vi "cameraSetup.vi"() -> ()   [LabVIEW 2024]
uses:
  <vilib>/userDefined/High Color/IMAQdx.ctl
  <vilib>/Python/Open Venv Python Session.vi
  <vilib>/vision/NI_Vision_Development_Module.lvlib
  <vilib>/vision/driver/NI_Vision_Acquisition_Software.lvlib
panel:
  out "Python Node Process Time":dbl
  out "error out":errorcluster
  out "PointCloud":T1(graph)=[{"appended array"=[-1.3170576278200137, -1.3344662442040491, -1.3432764589201578, -1.3444474689182773, -1.338872970131032, -1.327383409908652, -1.3107482394539027, -1.289678166257004, -1.26482740653056, -1.2367959376444793, -1.206131750560902, -1.1733331022691227, -1.1388507682205156, -1.1030902947634595, -1.0664142515782609, -1.0291444841120803, -0.9915643660138534, -0.9539210515692201, -0.9164277281354453, -0.879265868576345, -0.8425874836972105, -0.8065173746797322, -0.7711553855169254, -0.7365786554480533, -0.7028438713935529, -0.6699895203899575, -0.6380381420248239, -0.6069985808716541, -0.5768682389248215, -0.5476353280344943, -0.5192811223415612, -0.49178221071255507, -0.46511274917457684, -0.439246713350222, -0.41416015089250097, -0.38983343391976977, -0.3662535114506477, -0.34341616183894813, -0.3213282452085969, -0.300009955888562, -0.27949707484777436, -0.259843222130055, -0.2411221092890378, -0.22342979182309308, -0.2068869216102553, -0.19164099934314494, -0.17786862696389336, -0.16577776009906756, -0.15560996049459447, -0.14764264845068567], "appended array"=[0.03, 0.09530612244897953, 0.16061224489795906, 0.22591836734693857, 0.2912244897959181, 0.3565306122448982, 0.4218367346938777, 0.4871428571428572, 0.5524489795918368, 0.6177551020408163, 0.6830612244897958, 0.7483673469387756, 0.8136734693877551, 0.8789795918367347, 0.9442857142857145, 1.0095918367346939, 1.0748979591836736, 1.140204081632653, 1.2055102040816326, 1.2708163265306123, 1.336122448979592, 1.4014285714285715, 1.4667346938775512, 1.5320408163265307, 1.5973469387755104, 1.6626530612244899, 1.7279591836734693, 1.793265306122449, 1.8585714285714285, 1.9238775510204082, 1.989183673469388, 2.0544897959183674, 2.119795918367347, 2.1851020408163264, 2.250408163265306, 2.315714285714286, 2.3810204081632653, 2.446326530612245, 2.5116326530612247, 2.5769387755102042, 2.6422448979591837, 2.707551020408163, 2.7728571428571427, 2.838163265306122, 2.9034693877551025, 2.968775510204082, 3.0340816326530615, 3.099387755102041, 3.1646938775510205, 3.23]}, {"appended array"=[1.1959745945438647, 1.1539974976878962, 1.116034957811131, 1.081567752911547, 1.050122782354486, 1.021271082137672, 0.9946258401561943, 0.9698404114675151, 0.9466063335564582, 0.9246513416002126, 0.9037373837333251, 0.8836586363127031, 0.8642395191826058, 0.8453327109396446, 0.8268171641977818, 0.8085961208533234, 0.7905951273499227, 0.7727600499435693, 0.7550550899675955, 0.737460799097667, 0.7199720946167827, 0.702596274680272, 0.6853510335807903, 0.6682624770133202, 0.6513631373401643, 0.6346899888559443, 0.6182824630525999, 0.6021804638843833, 0.5864223830328587, 0.5710431151718984, 0.5560720732326803, 0.5415312036686851, 0.5274330017206939, 0.5137785266817849, 0.5005554171623322, 0.4877359063550006, 0.4752748372997456, 0.46310767814880766, 0.45114853743171296, 0.43928817932026787, 0.4273920388935579, 0.41529823740294264, 0.40281559753705665, 0.38972165868680464, 0.3757606922103577, 0.36064171669815265, 0.34403651323788836, 0.32557764067952294, 0.3048564509002722, 0.2814211040696046], "appended array"=[0.07, 0.13530612244897952, 0.20061224489795904, 0.2659183673469386, 0.3312244897959181, 0.39653061224489816, 0.4618367346938777, 0.5271428571428572, 0.5924489795918367, 0.6577551020408163, 0.7230612244897958, 0.7883673469387756, 0.8536734693877551, 0.9189795918367346, 0.9842857142857144, 1.049591836734694, 1.1148979591836736, 1.1802040816326531, 1.2455102040816326, 1.3108163265306123, 1.3761224489795918, 1.4414285714285715, 1.5067346938775512, 1.5720408163265307, 1.6373469387755102, 1.70265306122449, 1.7679591836734694, 1.833265306122449, 1.8985714285714286, 1.9638775510204083, 2.029183673469388, 2.0944897959183675, 2.159795918367347, 2.2251020408163265, 2.290408163265306, 2.355714285714286, 2.4210204081632654, 2.486326530612245, 2.5516326530612248, 2.6169387755102043, 2.6822448979591837, 2.7475510204081632, 2.8128571428571427, 2.878163265306122, 2.9434693877551026, 3.008775510204082, 3.0740816326530616, 3.139387755102041, 3.2046938775510205, 3.27]}, {"appended array"=[-2.1976754604858093, -2.1730091080730474, -2.147243328942704, -2.120370792552189, -2.0923975746039645, -2.063342224625402, -2.033234833548644, -2.002116101290463, -1.9700364043321177, -1.937054863299217, -1.903238410541575, -1.86866085771307, -1.8334019633515066, -1.7975465004584736, -1.7611833240791992, -1.7244044388824187, -1.687304066740224, -1.6499777143079288, -1.6125212406039253, -1.5750299245895452, -1.5375975327489153, -1.5003153866688206, -1.4632714306185601, -1.426549299129809, -1.3902273845764739, -1.3543779047545552, -1.3190659704620058, -1.284348653078588, -1.250274052145734, -1.216880362946406, -1.1841949440849537, -1.1522333850669733, -1.1209985738791681, -1.0904797645692061, -1.0606516448255798, -1.031473403557465, -1.0028877984745799, -0.9748202236670446, -0.9471777771852397, -0.9198483286196648, -0.8926995866807996, -0.8655781667789612, -0.8383086586041626, -0.810692693705974, -0.7825080130733804, -0.7535075347146409, -0.7234184212371477, -0.6919411474272857, -0.6587485678302909, -0.6234849843301098], "appended array"=[0.12, 0.18428571428571444, 0.24857142857142833, 0.3128571428571428, 0.3771428571428572, 0.44142857142857167, 0.5057142857142856, 0.5700000000000001, 0.6342857142857145, 0.698571428571429, 0.7628571428571428, 0.8271428571428573, 0.8914285714285715, 0.9557142857142855, 1.02, 1.0842857142857145, 1.1485714285714286, 1.2128571428571429, 1.2771428571428574, 1.3414285714285716, 1.405714285714286, 1.47, 1.5342857142857145, 1.5985714285714288, 1.6628571428571428, 1.7271428571428573, 1.7914285714285714, 1.8557142857142859, 1.92, 1.9842857142857144, 2.0485714285714285, 2.112857142857143, 2.1771428571428575, 2.2414285714285715, 2.305714285714286, 2.37, 2.4342857142857146, 2.4985714285714287, 2.5628571428571436, 2.6271428571428572, 2.6914285714285717, 2.755714285714286, 2.82, 2.8842857142857143, 2.948571428571429, 3.012857142857143, 3.0771428571428574, 3.141428571428572, 3.2057142857142855, 3.27]}, {"appended array"=[2.0462614612009418, 2.012322089098866, 1.9811875610569154, 1.9523916760385782, 1.9255095718547126, 1.9001560984615924, 1.8759841912589486, 1.8526832443880148, 1.8299774840295686, 1.8076243417019748, 1.7854128275592256, 1.7631619036889907, 1.7407188574106534, 1.7179576745733556, 1.6947774128540425, 1.6711005750555046, 1.646871482404418, 1.6220546478493925, 1.5966331493590098, 1.5706070032198705, 1.5439915373346338, 1.516815764520062, 1.4891207558050628, 1.4609580137287332, 1.4323878456384034, 1.4034777369876759, 1.3743007246344723, 1.3449337701390756, 1.315456133062171, 1.2859477442628913, 1.2564875791968586, 1.2271520312142292, 1.198013284857733, 1.1691376891607195, 1.140584130945199, 1.1124024081198882, 1.0846316029782503, 1.0572984554965381, 1.03041573663184, 1.003980621620119, 0.9779730632742587, 0.9523541652821047, 0.9270645555045082, 0.9020227592733693, 0.8771235726896788, 0.8522364359215618, 0.8272038065023218, 0.8018395326284821, 0.7759272264578283, 0.7492186374074544], "appended array"=[0.32, 0.380204081632653, 0.440408163265306, 0.5006122448979591, 0.5608163265306121, 0.6210204081632651, 0.6812244897959181, 0.7414285714285714, 0.8016326530612244, 0.8618367346938777, 0.9220408163265308, 0.9822448979591838, 1.0424489795918368, 1.1026530612244898, 1.1628571428571428, 1.2230612244897958, 1.2832653061224488, 1.3434693877551018, 1.403673469387755, 1.463877551020408, 1.5240816326530613, 1.5842857142857145, 1.6444897959183673, 1.7046938775510205, 1.7648979591836735, 1.8251020408163265, 1.8853061224489795, 1.9455102040816326, 2.005714285714286, 2.065918367346939, 2.126122448979592, 2.186326530612245, 2.246530612244898, 2.306734693877551, 2.366938775510204, 2.427142857142857, 2.4873469387755103, 2.5475510204081635, 2.6077551020408163, 2.6679591836734695, 2.7281632653061223, 2.7883673469387755, 2.8485714285714288, 2.9087755102040815, 2.9689795918367343, 3.029183673469388, 3.089387755102041, 3.149591836734694, 3.2097959183673472, 3.27]}]
  out "Image":T2(plugin-control)
  out "yellow_right_y":dbl[](array[numeric])
  out "yellow_right_x":dbl[](array[numeric])
  out "yellow_left_y":dbl[](array[numeric])
  out "yellow_left_x":dbl[](array[numeric])
  out "white_right_y":dbl[](array[numeric])
  out "white_right_x":dbl[](array[numeric])
  out "white_left_y":dbl[](array[numeric])
  out "white_left_x":dbl[](array[numeric])
  in  "Test":bool=TRUE
  in  "Cam No.":T3
  out "Python Loop Process Time":u32=101
  out "B Pixels":u8[][](array[numeric])
  out "G Pixels":u8[][](array[numeric])
  out "R Pixels":u8[][](array[numeric])
  out "Image2Array LoopTime":u32=101
  in  "stop":bool
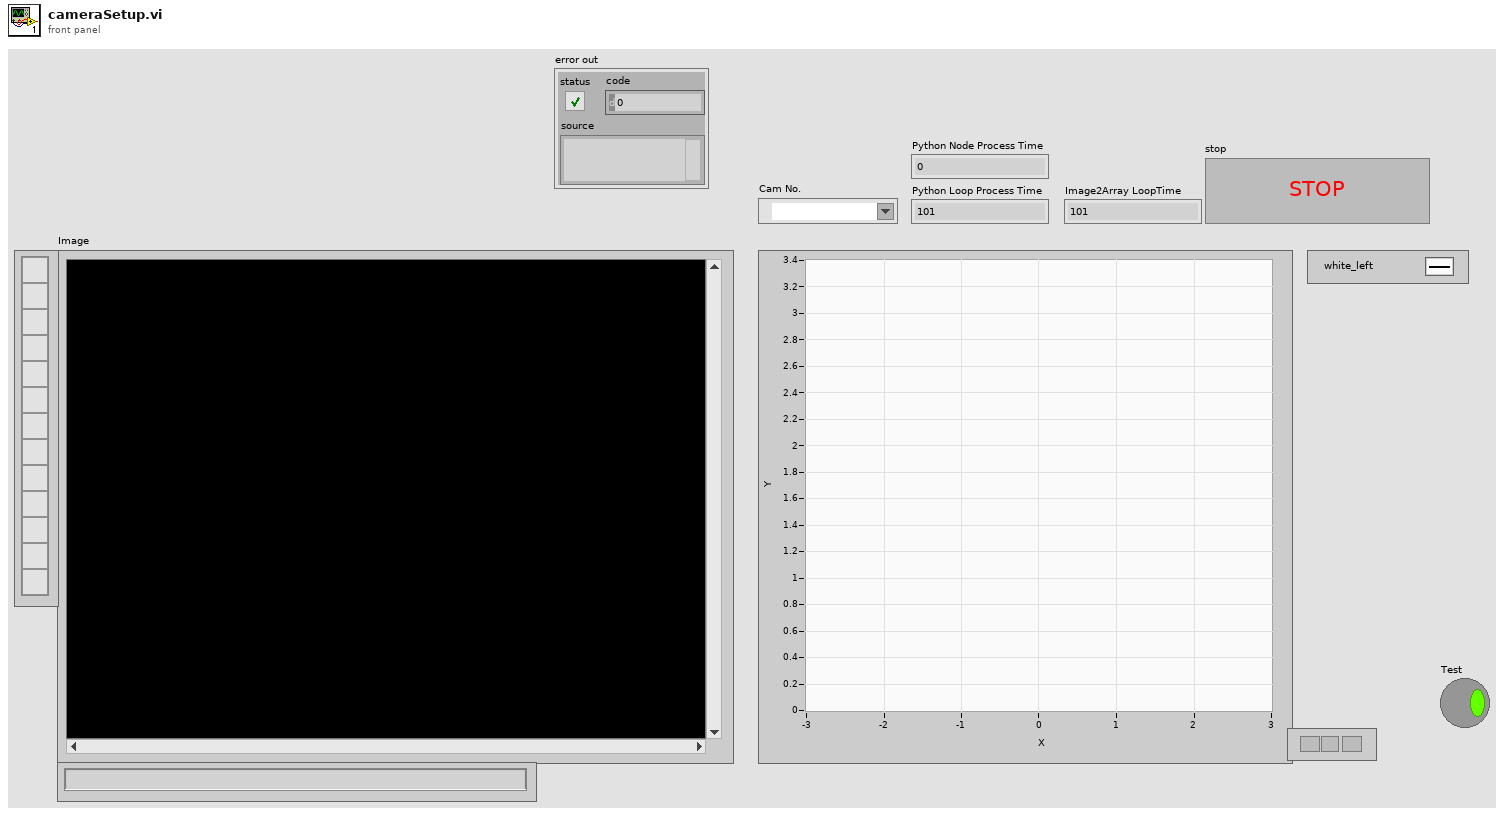
[diagram p1: front panel]
types:
  T1 = cluster{"appended array":dbl[], "appended array":dbl[]}[]
  T2 = typedef "IMAQ Image.ctl" = refnum<image>
  T3 = typedef "IMAQdx.ctl" = refnum<k21>
  T4 = cluster{"white_left_x":dbl[], "white_left_y":dbl[]}
  T5 = cluster{"white_right_x":dbl[], "white_right_y":dbl[]}
  T6 = cluster{"yellow_left_x":dbl[], "yellow_left_y":dbl[]}
  T7 = cluster{"yellow_right_x":dbl[], "yellow_right_y":dbl[]}
  T8 = cluster{"yellow_right_x":dbl[], "yellow_right_y":dbl[]}[]
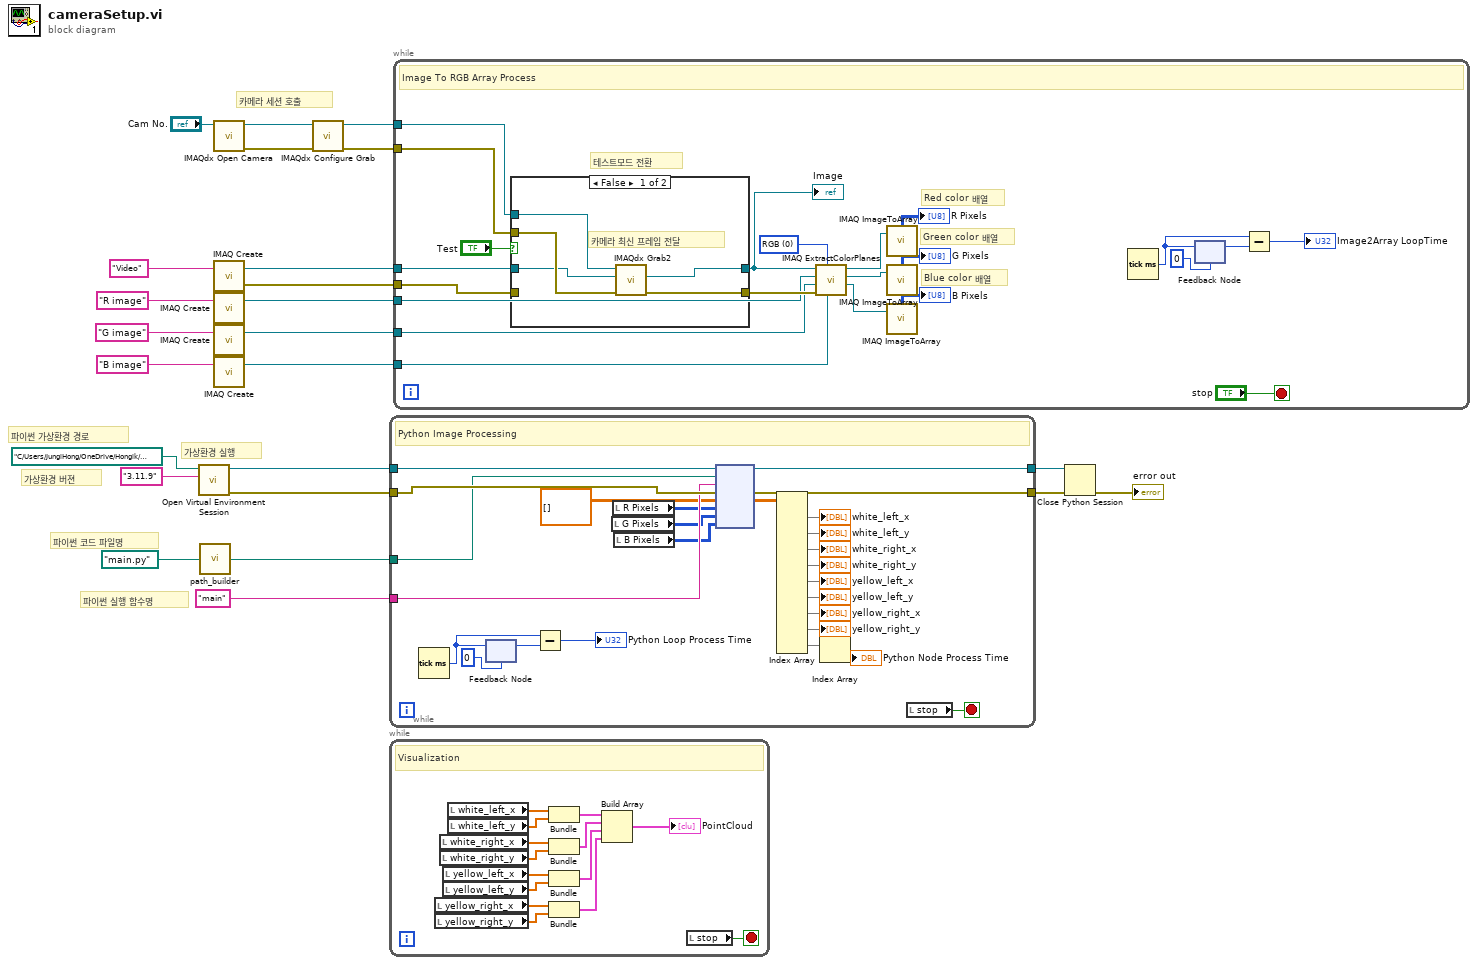
[diagram p0: block diagram]
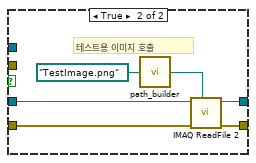
[diagram p2: hidden frame]
diagram:
  # "파이썬 실행 함수명"
  # "파이썬 코드 파일명"
  # "가상환경 실행"
  # "가상환경 버젼"
  # "파이썬 가상환경 경로"
  # "카메라 세션 호출"
  n1 = call-poly <vilib>:"Open Virtual Environment Session.vi"("Python version"="3.11.9", "Env path"=path "C:/Users/JungiHong/OneDrive/Hongik/HI-RACE/2026-01/.venv") -> ("error out"=w10:errorcluster, "session out"=w11:refnum<k35>)  [unwired: 8 in]
  n2 = call "path_builder.vi"("Name"=path "main.py") -> ("appended path"=w9:path)
  n3 = call <vilib>:"IMAQdx Open Camera.vi"("Session In"="Cam No.") -> ("error out"=w5:errorcluster, "Session Out"=w6:T3)  [unwired: 9 in]
  n4 = call "IMAQ Create"("Image Name"="Video") -> ("New Image"=w20:T2, "error out"=w21:errorcluster)  [unwired: 4 in]
  n5 = call "IMAQ Create"("Image Name"="R image") -> ("New Image"=w16:T2)  [unwired: 4 in, 1 out]
  n6 = call "IMAQ Create"("Image Name"="G image") -> ("New Image"=w15:T2)  [unwired: 4 in, 1 out]
  n7 = call "IMAQ Create"("Image Name"="B image") -> ("New Image"=w14:T2)  [unwired: 4 in, 1 out]
  n8 = call <vilib>:"IMAQdx Configure Grab.vi"("error in"=w5, "Session In"=w6) -> ("error out"=w2:errorcluster, "Session Out"=w3:T3)  [unwired: 8 in]
  n9 = while {
    tunnel: w9 -> [w46]
    tunnel: "main" ("module out") -> [w45]
    tunnel: w11 -> [w48]
    tunnel: [w50] -> w13
    tunnel: w10 -> [w47]
    tunnel: [w49] -> w12
    stop <- w41 stop-if-true
    # "Python Image Processing"
    n10 = Tick Count (ms)() -> (millisecond timer value=w37:u32)
    n11 = feedback #1(u32 0 ("millisecond timer value")) -> (w38:u32)
    n12 = feedback-in #1(w37) -> ()
    n13 = Subtract(x=w37, y=w38) -> (x-y=→"Python Loop Process Time":u32)
    n14 = local read "G Pixels"() -> (w43:u8[][])
    n15 = local read "R Pixels"() -> (w44:u8[][])
    n16 = local read "B Pixels"() -> (w42:u8[][])
    n17 = node(w48, w46, w45, w47, dbl[][] [] ("appended array"), w44, w43, w42) -> (w50:refnum<k35>, w49:errorcluster, w35:dbl[][])  [unwired: 3 in, 2 out]
    n18 = Index Array(array=w35) -> (element #1=→"white_left_x":dbl[], element #2=→"white_left_y":dbl[], element #3=→"white_right_x":dbl[], element #4=→"white_right_y":dbl[], element #5=→"yellow_left_x":dbl[], element #6=→"yellow_left_y":dbl[], element #7=→"yellow_right_x":dbl[], element #8=→"yellow_right_y":dbl[], element #9=w26:dbl[])  [unwired: 18 in]
    n19 = Index Array(array=w26) -> (element=→"Python Node Process Time":dbl)  [unwired: 1 in]
    n20 = local read "stop"() -> (w41:bool)
  }
  n21 = while {
    stop <- w60 stop-if-true
    # "Visualization"
    n22 = local read "yellow_right_x"() -> (w52:dbl[])
    n23 = local read "yellow_right_y"() -> (w51:dbl[])
    n24 = local read "white_right_x"() -> (w56:dbl[])
    n25 = local read "white_right_y"() -> (w55:dbl[])
    n26 = local read "yellow_left_x"() -> (w54:dbl[])
    n27 = local read "yellow_left_y"() -> (w53:dbl[])
    n28 = local read "white_left_x"() -> (w58:dbl[])
    n29 = local read "white_left_y"() -> (w57:dbl[])
    n30 = Bundle("white_left_x"=w58, "white_left_y"=w57) -> (w64:T4)  [unwired: 1 in]
    n31 = Bundle("white_right_x"=w56, "white_right_y"=w55) -> (w63:T5)  [unwired: 1 in]
    n32 = Bundle("yellow_left_x"=w54, "yellow_left_y"=w53) -> (w62:T6)  [unwired: 1 in]
    n33 = Bundle("yellow_right_x"=w52, "yellow_right_y"=w51) -> (w61:T7)  [unwired: 1 in]
    n34 = Build Array(w64, w63, w62, w61) -> (→"PointCloud":T8)
    n35 = local read "stop"() -> (w60:bool)
  }
  n36 = while {
    tunnel: w21 -> [w82]
    tunnel: w20 -> [w81]
    tunnel: w16 -> [w79]
    tunnel: w15 -> [w78]
    tunnel: w14 -> [w77]
    tunnel: w3 -> [w66]
    tunnel: w2 -> [w67]
    stop <- "stop" stop-if-true
    w86 = u16 0 items=["RGB", "HSL", "HSV", "HSI"] ("Color Mode")
    # "Blue color 배열"
    # "Green color 배열"
    # "Red color 배열"
    # "테스트모드 전환"
    # "Image To RGB Array Process"
    n37 = case shown="False" "Test" {
      tunnel: w82 -> [_ w97]
      tunnel: w81 -> [w87 w96]
      tunnel: [w88 w95] -> w80
      tunnel: [w89 w94] -> w65
      tunnel: w67 -> [w91 _]
      tunnel: w66 -> [w90 _]
      frame False {
        # "카메라 최신 프레임 전달"
        n38 = call <vilib>:"IMAQdx Grab2.vi"("error in"=w91, "Image In"=w87, "Session In"=w90) -> ("error out"=w88:errorcluster, "Image Out"=w89:T2)  [unwired: 5 in, 2 out]
      }
      frame True {
        # "테스트용 이미지 호출"
        n39 = call "path_builder.vi"("Name"=path "TestImage.png") -> ("appended path"=w93:path)
        n40 = call "IMAQ ReadFile 2"("File Path"=w93, "error in (no error)"=w97, "Image"=w96) -> ("error out"=w95:errorcluster, "Image Out"=w94:T2)  [unwired: 4 in, 3 out]
      }
    }
    "Image" <- w65
    n41 = call "IMAQ ExtractColorPlanes"("Blue or Luma or Val or Inten Plane"=w77, "Color Mode"=w86, "error in (no error)"=w80, "Green or Sat Plane"=w78, "Red or Hue Plane"=w79, "Image Src"=w65) -> ("Blue or Luma or Val or Inten Plane out"=w83:T2, "Green or Sat Plane out"=w84:T2, "Red or Hue Plane out"=w85:T2)  [unwired: 2 in, 1 out]
    n42 = call "IMAQ ImageToArray"("Image"=w85) -> ("Image Pixels (U8)"=→"R Pixels":u8[][])  [unwired: 3 in, 4 out]
    n43 = call "IMAQ ImageToArray"("Image"=w84) -> ("Image Pixels (U8)"=→"G Pixels":u8[][])  [unwired: 3 in, 4 out]
    n44 = call "IMAQ ImageToArray"("Image"=w83) -> ("Image Pixels (U8)"=→"B Pixels":u8[][])  [unwired: 3 in, 4 out]
    n45 = Tick Count (ms)() -> (millisecond timer value=w76:u32)
    n46 = feedback #2(u32 0 ("millisecond timer value")) -> (w75:u32)
    n47 = feedback-in #2(w76) -> ()
    n48 = Subtract(x=w76, y=w75) -> (x-y=→"Image2Array LoopTime":u32)
  }
  n49 = Close Python Session(session in=w13, error in=w12) -> (11:→"error out":errorcluster)
